vi "ArmCheckOnTarget.vi"(9 "Desired Extend (inch)":dbl, 11 "Desired Lift (deg)":dbl) -> (3 "On Target":bool)   [LabVIEW 2020]
doc: "Get current position\n\nOutput:\n--RotatePosition -- Double -- Degrees\n--LiftPosition -- Double -- Degrees\n--ExtendPosition -- Double -- Inches"
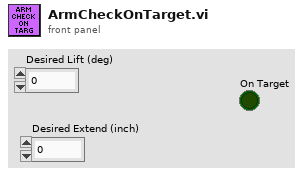
[diagram p1: front panel]
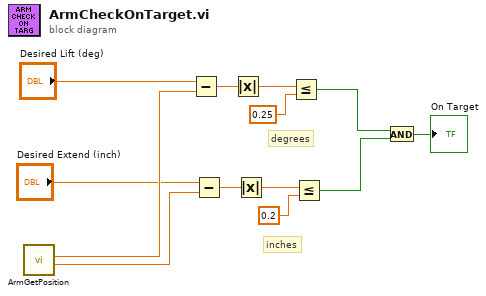
[diagram p0: block diagram]
diagram:
  # "degrees"
  # "inches"
  n1 = call "ArmGetPosition.vi"() -> ("ExtendPostion"=w6:dbl, "LiftPostion"=w7:dbl)  [unwired: 10 in]
  n2 = Subtract(x="Desired Lift (deg)", y=w7) -> (x-y=w13:dbl)
  n3 = Subtract(x="Desired Extend (inch)", y=w6) -> (x-y=w10:dbl)
  n4 = Absolute Value(x=w13) -> (abs(x)=w12:dbl)
  n5 = Absolute Value(x=w10) -> (abs(x)=w9:dbl)
  n6 = Less Or Equal?(x=w12, y=0.25) -> (x <= y?=w3:bool)
  n7 = Less Or Equal?(x=w9, y=0.2) -> (x <= y?=w2:bool)
  n8 = And(x=w3, y=w2) -> (x .and. y?=→"On Target":bool)
